vi "Configure Triggered Voltage Level [TRG] Core.vi"(8 "error in (no error)":errorcluster, 9 "triggered level (0.0 Volts)":dbl[unit] format="%^.2e", 10 "channel name (\"CHANNEL1\")":string="CHANNEL1", 11 "IVI_DCPwr in":refnum<class "IVI_DCPwr.lvclass">) -> (0 "error out":errorcluster, 3 "IVI_DCPwr out":refnum<class "IVI_DCPwr.lvclass">)   [LabVIEW 2015, in "IVI_DCPwr.lvlib" / "IVI_DCPwr.lvclass"]
doc: "This VI configures the DC voltage level the power supply attempts to generate after it receives a trigger.\n\nNotes:\n\n(1) This VI is part of the IviDCPwrTrigger [TRG] extension group."
uses:
  IVI_DCPwr.lvclass
  IVI_DCPwr.lvclass/IVI_DCPwr.ctl
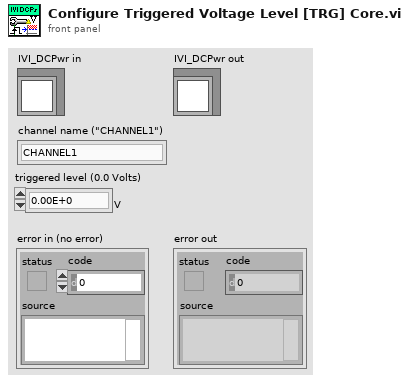
[diagram p1: front panel]
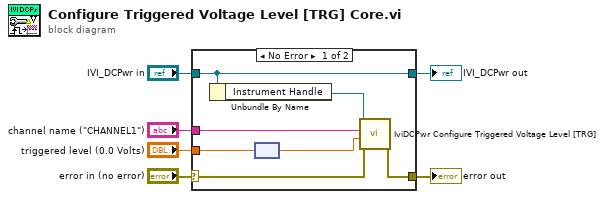
[diagram p0: block diagram]
diagram:
  n1 = case shown="No Error" "error in (no error)" {
    selector: "error in (no error)" -> [w11 w15]
    tunnel: [w10 w15] -> w5
    tunnel: [w13 w14] -> w3
    tunnel: "IVI_DCPwr in" -> [w13 w14]
    tunnel: "channel name (\"CHANNEL1\")" -> [w9 _]
    tunnel: "triggered level (0.0 Volts)" -> [w8 _]
    frame No Error {
      n2 = Unbundle By Name(w13) -> ("Instrument Handle"=w12:refnum<k15>)
      n3 = node(w8) -> (w7:dbl)
      n4 = call <vilib>:"IviDCPwr Configure Triggered Voltage Level [TRG].vi"("error in (no error)"=w11, "triggered level (0.0 Volts)"=w7, "channel name (\"CHANNEL1\")"=w9, "instrument handle"=w12) -> ("error out"=w10:errorcluster)  [unwired: 6 in, 1 out]
    }
    frame Error {
    }
  }
  "error out" <- w5
  "IVI_DCPwr out" <- w3
